vi "Build Signals.vi"(5 "WCM_corrections":bool, 7 "WCM_values":sgl[](array[numeric]), 8 "error in (no error)":errorcluster, 9 "II channel seq":cluster{"BG":i32[], "Ie":i32[], "I0":i32[]}[](array[cluster]), 10 "I channel seq":cluster{"BG":i32[], "Ie":i32[], "I0":i32[]}[](array[cluster]), 11 "VIS-IR in":refnum<class "VIS-IR.lvclass">) -> (0 "error out":errorcluster, 1 "Signals so Send":T1, 2 "Signals":cluster{"wavelengths":dbl[], "Tableau":dbl[]}[](array[cluster]), 3 "VIS-IR out":refnum<class "VIS-IR.lvclass">, 4 "#PP":i32)   [LabVIEW 2015, in "VIS-IR.lvclass"]
uses:
  VIS-IR.lvclass
  dependecies/ControlsVIs/Clusters-def/Def_signals_from_DET.ctl
  Detector.lvclass
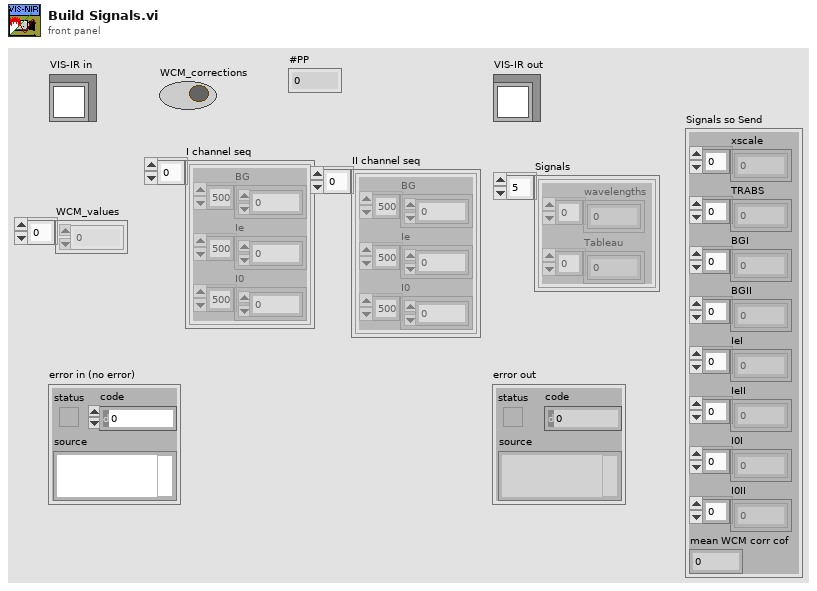
[diagram p1: front panel]
types:
  T1 = typedef "Def_signals_from_DET.ctl" = cluster{"xscale":dbl[], "TRABS":dbl[], "BGI":i32[], "BGII":i32[], "IeI":i32[], "IeII":i32[], "I0I":i32[], "I0II":i32[], "mean WCM corr cof":dbl}
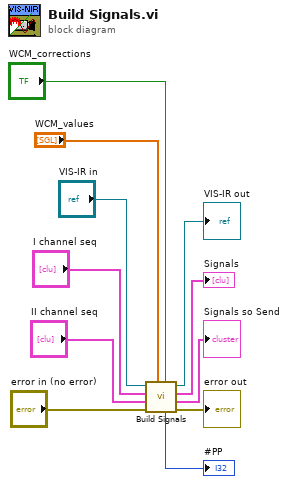
[diagram p0: block diagram]
diagram:
  n1 = call-parent "Build Signals.vi"("WCM_corrections"="WCM_corrections", "WCM_values"="WCM_values", "error in (no error)"="error in (no error)", "II channel seq"="II channel seq", "I channel seq"="I channel seq", "Detector in"="VIS-IR in") -> ("error out"=→"error out":errorcluster, "Signals so Send"=→"Signals so Send":T1, "Signals"=→"Signals":cluster{"wavelengths":dbl[], "Tableau":dbl[]}[], "Detector out"=→"VIS-IR out":refnum<class "VIS-IR.lvclass">, "#PP"=→"#PP":i32)  [unwired: 1 in]
